vi "move-motor_RL.vi"(8 "error in":errorcluster, 11 "Direction":bool) -> (0 "error out":errorcluster, 3 "Current Stepp":i32)   [LabVIEW 2021]
doc: "Random Laser Project v2.0\nAndré Romero - 2024\nandretec@ifsc.usp.br"
uses:
  Global_v20.vi
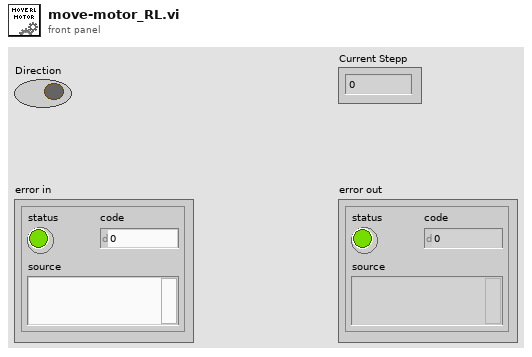
[diagram p1: front panel]
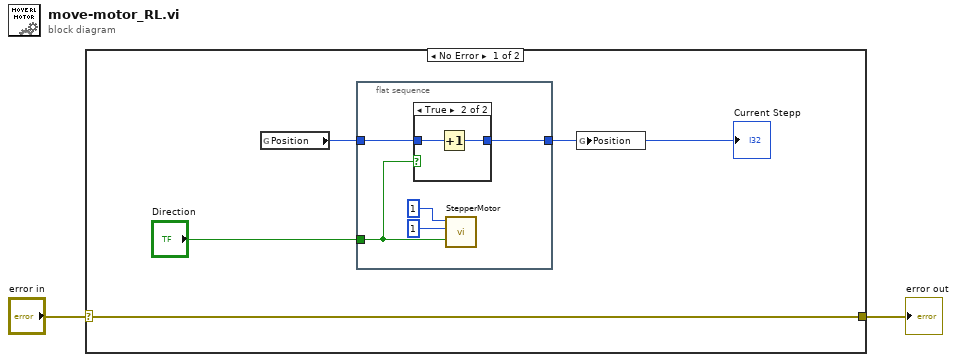
[diagram p0: block diagram]
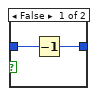
[diagram p2: hidden frame]
diagram:
  n1 = case shown="No Error" "error in" {
    selector: "error in" -> [w3 w16]
    tunnel: [w3 w16] -> w1
    frame No Error {
      n2 = global read "Global_v20.vi" "Position"() -> (w4:i32)
      n3 = flat-sequence {
        tunnel: w4 -> [w9]
        tunnel: [w8] -> w5
        tunnel: "Direction" -> [w7]
        frame #0 {
          n4 = case shown="True" w7 {
            tunnel: w9 -> [w13 w15]
            tunnel: [w12 w14] -> w8
            frame False {
              n5 = Decrement(x=w13) -> (x-1=w12:i32)
            }
            frame True {
              n6 = Increment(x=w15) -> (x+1=w14:i32)
            }
          }
          n7 = call "StepperMotor.vi"("Direction"=w7, "Time between steps (ms)"=1, "Steps"=i64 1) -> ()  [unwired: 8 in, 1 out]
        }
      }
      n8 = global write "Global_v20.vi" "Position"(w5) -> ()
      "Current Stepp" <- w5
    }
    frame Error {
    }
  }
  "error out" <- w1
